vi "checkTimeout.vi"(8 "error in (no error)":errorcluster, 10 "executionTime":dbl, 11 "Monochromator in":refnum<class "Monochromator.lvclass">) -> (0 "error out":errorcluster, 2 "timeout":bool, 3 "Monochromator out":refnum<class "Monochromator.lvclass">)   [LabVIEW 2016, in "Monochromator.lvclass"]
uses:
  Monochromator.lvclass
  Monochromator.lvclass/Monochromator.ctl
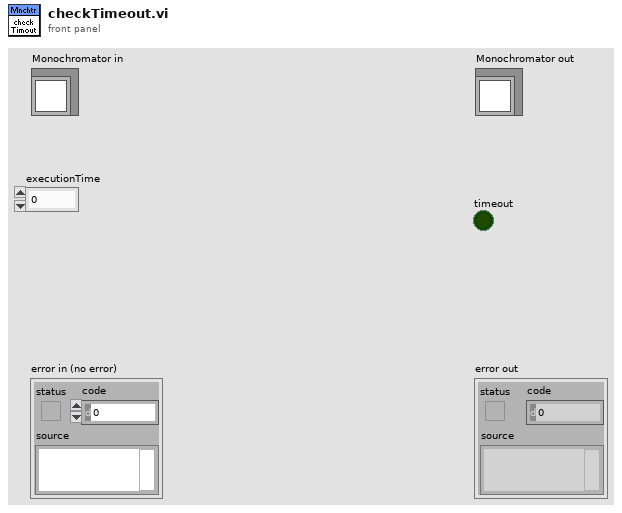
[diagram p1: front panel]
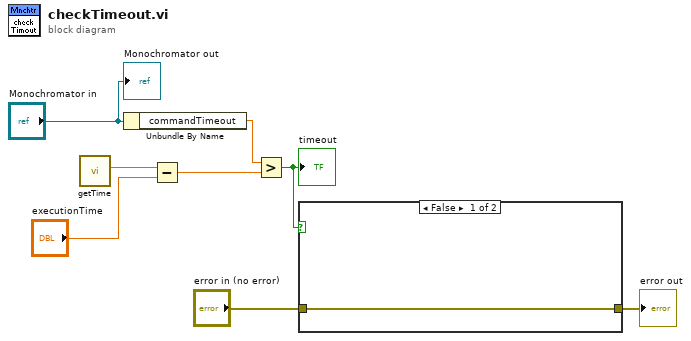
[diagram p0: block diagram]
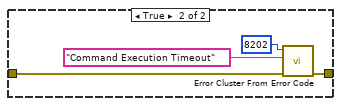
[diagram p2: hidden frame]
diagram:
  n1 = call "getTime.vi"() -> ("timestamp"=w6:dbl)  [unwired: 9 in, 2 out]
  n2 = Unbundle By Name("Monochromator in") -> ("commandTimeout"=w7:dbl)
  n3 = Subtract(x=w6, y="executionTime") -> (x-y=w4:dbl)
  n4 = Greater?(x=w7, y=w4) -> (0:w3:bool)
  "timeout" <- w3
  n5 = case shown="False" w3 {
    tunnel: "error in (no error)" -> [w9 w13]
    tunnel: [w9 w12] -> w1
    frame False {
    }
    frame True {
      n6 = call <vilib>:"Error Cluster From Error Code.vi"("error in (no error)"=w13, "error message (\"\")"="Command Execution Timeout" ("error message (\"\")"), "error code (0)"=8202) -> ("error out"=w12:errorcluster)  [unwired: 6 in]
    }
  }
  "error out" <- w1
  "Monochromator out" <- "Monochromator in"
